vi "RedEdge Manager.vi"(8 "error in (no error)":errorcluster) -> ()   [LabVIEW 2014]
uses:
  Controls/RedEdge Status.ctl
  Application Support/Stop Button/SubVI/Get Stop Button Status.vi
  <vilib>/httpClient/LabVIEWHTTPClient.lvlib
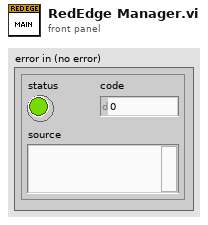
[diagram p1: front panel]
types:
  T1 = typedef "RedEdge Status.ctl" = cluster{"alt_agl":dbl, "auto_cap_active":bool, "bus_volts":i32, "course":i32, "gps_lat":dbl, "gps_time":string, "gps_used_sats":i32, "gps_vis_sats":i32, "gps_warn":bool, "p_acc":i32, "sd_gb_free":i32, "sd_gb_total":i32, "sd_status":string, "sd_warn":bool, "sv_info":cluster{"azimuth":i32, "channel":i32, "cno":i32, "diff_flag":bool, "elevation":i32, "orbit_info":bool, "orbit_is_eph":bool, "quality":i32, "sv_healthy":bool, "svid":i32, "used_flag":bool}[], "utc_time":string, "vel_2d":i32}
  T2 = typedef "LabVIEWHTTPClient.lvlib/ClientHandle.ctl" = refnum<k1>
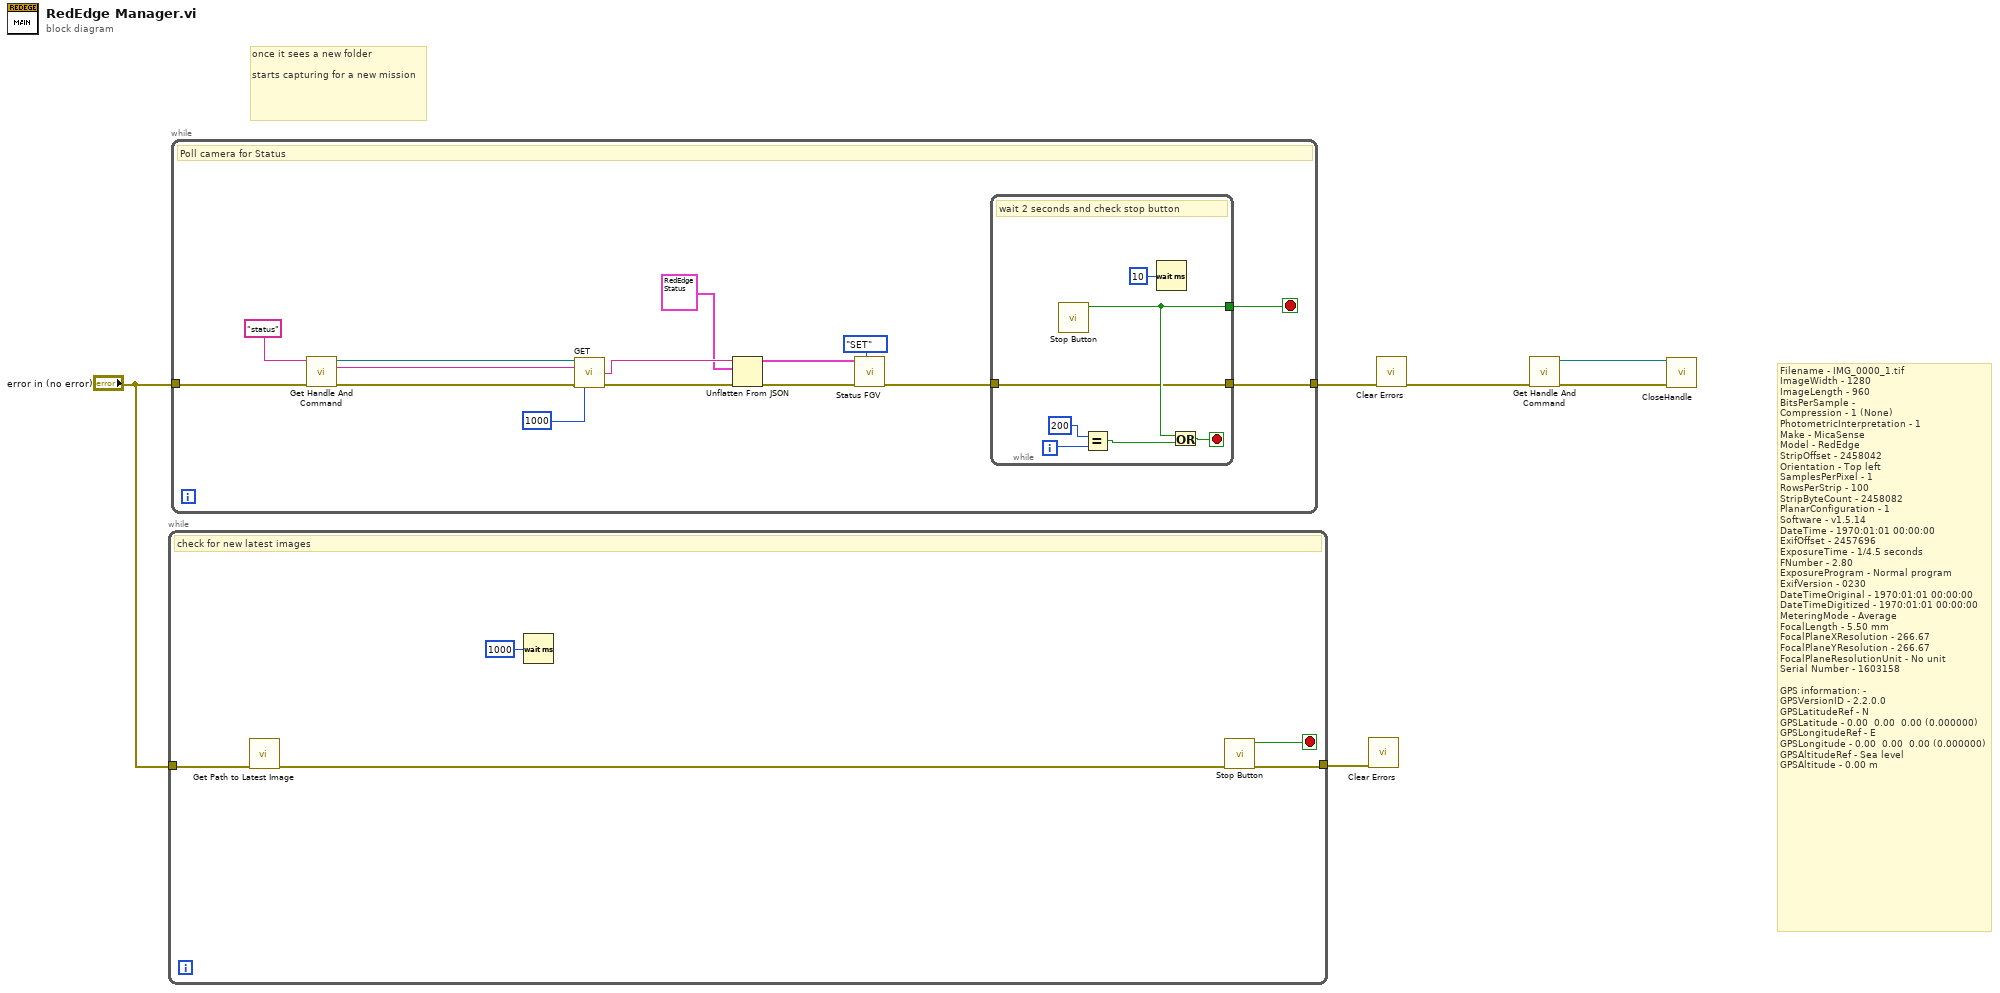
[diagram p0: block diagram]
diagram:
  # "once it sees a new folder\n\nstarts capturing for a new mission"
  # "Filename - IMG_0000_1.tif\nImageWidth - 1280\nImageLength - 960\nBitsPerSample - \nCompression - 1 (None)\nPhotometricInterpretation - 1\nMake - MicaSense\nModel - RedEdge\nStripOffset - 2458042\nOrientation - Top left\nSamplesPerPixel - 1\nRowsPerStrip - 100\nStripByteCount - 2458082\nPlanarConfiguration - 1\nSoftware - v1.5.14\nDateTime - 1970:01:01 00:00:00\nExifOffset - 2457696\nExposureTime - 1/4.5 seconds\nFNumber - 2.80\nExposureProgram - Normal program\nExifVersion - 0230\nDateTimeOriginal - 1970:01:01 00:00:00\nDateTimeDigitized - 1970:01:01 00:00:00\nMeteringMode - Average\nFocalLength - 5.50 mm\nFocalPlaneXResolution - 266.67\nFocalPlaneYResolution - 266.67\nFocalPlaneResolutionUnit - No unit\nSerial Number - 1603158\n\nGPS information: - \nGPSVersionID - 2.2.0.0\nGPSLatitudeRef - N\nGPSLatitude - 0.00  0.00  0.00 (0.000000)\nGPSLongitudeRef - E\nGPSLongitude - 0.00  0.00  0.00 (0.000000)\nGPSAltitudeRef - Sea level\nGPSAltitude - 0.00 m"
  n1 = while {
    tunnel: "error in (no error)" -> [w11]
    tunnel: [w9] -> w1
    stop <- w10 stop-if-true
    # "check for new latest images"
    n2 = call "Get Path to Latest Image.vi"("Error In"=w11) -> ("error out"=w7:errorcluster)  [unwired: 9 in, 1 out]
    n3 = Wait (ms)(milliseconds to wait=u32 1000) -> ()  [unwired: 1 out]
    n4 = call-poly "Stop Button.vi"("Error In"=w7) -> ("Error Out"=w9:errorcluster, "Stop ButtonOut"=w10:bool)  [unwired: 9 in]
  }
  n5 = while {
    tunnel: [w12] -> w6
    tunnel: "error in (no error)" -> [w17]
    stop <- w15 stop-if-true
    # "Poll camera for Status"
    n6 = call "Get Handle And Command.vi"("Error In"=w17, "Command"="status" ("string")) -> ("Error Out"=w19:errorcluster, "Command URL"=w16:string, "RedEdge client handle out"=w20:T2)  [unwired: 6 in]
    n7 = call <vilib>:"GET.vi"("client handle"=w20, "url"=w16, "error in (no error)"=w19, "timeout (10000)"=1000) -> ("body"=w26:string, "error out"=w21:errorcluster)  [unwired: 8 in, 2 out]
    n8 = Unflatten From JSON(JSON string=w26, type and defaults=T1 {"alt_agl"=0.0, "auto_cap_active"=FALSE, "bus_volts"=0, "course"=0, "gps_lat"=0.0, "gps_time"="", "gps_used_sats"=0, "gps_vis_sats"=0, "gps_warn"=FALSE, "p_acc"=0, "sd_gb_free"=0, "sd_gb_total"=0, "sd_status"="", "sd_warn"=FALSE, "sv_info"=[], "utc_time"="", "vel_2d"=0} ("RedEdge Status"), error in (no error)=w21) -> (value=w23:T1, error out=w22:errorcluster)  [unwired: 4 in]
    n9 = call "Status FGV.vi"("Operation"=enum16{"GET", "SET"}."SET", "Error In"=w22, "Red Edge Status In"=w23) -> ("Error Out"=w13:errorcluster)  [unwired: 7 in, 1 out]
    n10 = while {
      tunnel: [w29] -> w15
      tunnel: w13 -> [w27]
      tunnel: [w27] -> w12
      i -> [w32]
      stop <- w28 stop-if-true
      # "wait 2 seconds and check stop button"
      n11 = call-poly "Stop Button.vi"() -> ("Stop ButtonOut"=w29:bool)  [unwired: 10 in, 1 out]
      n12 = Equal?(x=200, y=w32) -> (x = y?=w30:bool)
      n13 = Wait (ms)(milliseconds to wait=u32 10) -> ()  [unwired: 1 out]
      n14 = Or(x=w29, y=w30) -> (x .or. y?=w28:bool)
    }
  }
  n15 = call <vilib>:"Clear Errors.vi"("error in (no error)"=w1) -> ()  [unwired: 5 in, 2 out]
  n16 = call <vilib>:"Clear Errors.vi"("error in (no error)"=w6) -> ("error out"=w2:errorcluster)  [unwired: 5 in, 1 out]
  n17 = call "Get Handle And Command.vi"("Error In"=w2) -> ("Error Out"=w5:errorcluster, "RedEdge client handle out"=w4:T2)  [unwired: 7 in, 1 out]
  n18 = call <vilib>:"CloseHandle.vi"("client handle"=w4, "error in (no error)"=w5) -> ()  [unwired: 13 in, 1 out]
